vi "Recall Channel Coefficient.vi"(8 "error in (no error)":errorcluster, 10 "Memory Register (0: A)":i32(ring) items=["A", "B", "C", "D"], 11 "VISA resource name":refnum<visa-resource-name>) -> (0 "error out":errorcluster, 3 "VISA resource name out":refnum<visa-resource-name>)   [LabVIEW 2011, in "Agilent ENA Series.lvlib"]
doc: "Recalls the calibration coefficient for an individual channel from the specified register as the setting of the active channel.\n\nNotes:\n(1) It is possible to recall the register from a different channel where it was saved.\n(2) This VI is available only for ENA E5061A/E5062A."
uses:
  Agilent ENA Series.lvlib
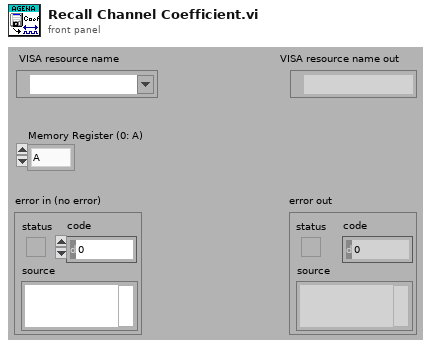
[diagram p1: front panel]
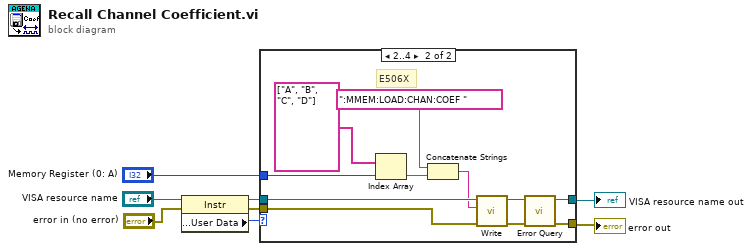
[diagram p0: block diagram]
diagram:
  n1 = property class="Instr"(reference="VISA resource name", error in="error in (no error)") -> (reference out=w8:refnum<visa-resource-name>, error out=w7:errorcluster, "General Settings:User Data"=w6:u32)
  n2 = case shown="2..4" w6 {
    tunnel: w8 -> [w10 w21]
    tunnel: w7 -> [w9 w20]
    tunnel: [w10 w12] -> w2
    tunnel: [w9 w11] -> w1
    tunnel: "Memory Register (0: A)" -> [_ w18]
    frame 0, Default {
    }
    frame 2..4 {
      # "E506X"
      n3 = Index Array(array=string[] ["A", "B", "C", "D"], index=w18) -> (element=w17:string)
      n4 = Concatenate Strings(":MMEM:LOAD:CHAN:COEF ", w17) -> (w15:string)
      n5 = call "Write.vi"("error in (no error)"=w20, "String ()"=w15, "VISA resource name"=w21) -> ("error out"=w13:errorcluster, "VISA resource name out"=w14:refnum<visa-resource-name>)  [unwired: 6 in, 1 out]
      n6 = call "Error Query.vi"("error in (no error)"=w13, "VISA resource name"=w14) -> ("error out"=w11:errorcluster, "VISA resource name out"=w12:refnum<visa-resource-name>)  [unwired: 6 in, 2 out]
    }
  }
  "error out" <- w1
  "VISA resource name out" <- w2
